vi "ActorDB-CheckIfPartExists.vi"(7 "Request Body":string, 8 "error in":errorcluster, 11 "Database-Actor in":refnum<class "PartCertDatabase-Actor.lvclass">) -> (0 "error out":errorcluster, 2 "Part number not found?":bool, 3 "Database-Actor out":refnum<class "PartCertDatabase-Actor.lvclass">)   [LabVIEW 2013, in "PartCertDatabase-Actor.lvclass"]
uses:
  PartCertDatabase-Actor.lvclass
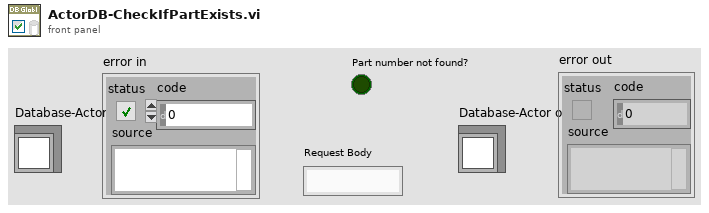
[diagram p1: front panel]
types:
  T1 = cluster{"Table":string, "SQL Statement":string, "Update All":bool, "Payload":string, "Reply Command":string, "Type Of Insertion":i32}
  T2 = cluster{"Manufacturing-Part Number":string, "Array of Cluster Data":cluster{"Label Instructions":string, "Path for Picture Label":path, "Path for Picture Label 2":path, "Path for Picture Label 3":path, "Path for Picture Label 4":path, "Path for Picture Label 5":path, "Path for Picture Label 6":path, "Path for Picture Label 7":path, "Label Instructions 2":string, "Label Instructions 3":string}[], "Type of Insert":i32}
  T3 = cluster{"Manufacturing-Part Number":string, "Step Number":dbl, "Gernal Cluster Data":cluster{"Label Instructions":string, "Path for Picture Label":path, "Path for Picture Label 2":path, "Path for Picture Label 3":path, "Path for Picture Label 4":path, "Path for Picture Label 5":path, "Path for Picture Label 6":path, "Path for Picture Label 7":path}, "Type of Insert":i32}
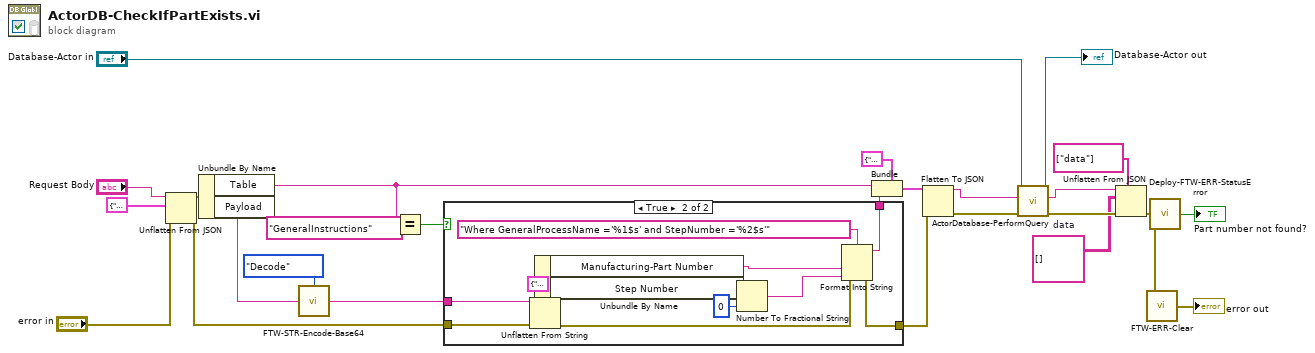
[diagram p0: block diagram]
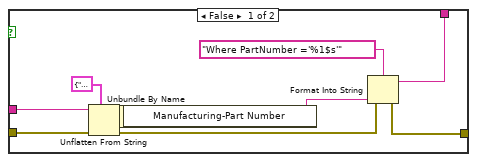
[diagram p2: hidden frame]
diagram:
  w7 = string[][] []  # data
  n1 = Unflatten From JSON(JSON string="Request Body", type and defaults=T1 {"Table"="", "SQL Statement"="", "Update All"=FALSE, "Payload"="", "Reply Command"="", "Type Of Insertion"=0} ("cluster"), error in (no error)="error in") -> (value=w23:T1, error out=w12:errorcluster)  [unwired: 4 in]
  n2 = Unbundle By Name(w23) -> ("Table"=w2:string, "Payload"=w21:string)
  n3 = call "FTW-STR-Encode-Base64.vi"("Input"=w21, "Direction"=enum16{"Encode", "Decode"}."Decode") -> ("Output"=w20:string)
  n4 = Equal?(x=w2, y="GeneralInstructions") -> (x = y?=w1:bool)
  n5 = case shown="True" w1 {
    tunnel: w20 -> [w35 w38]
    tunnel: [w30 w39] -> w17
    tunnel: [w29 w40] -> w16
    tunnel: w12 -> [w28 w41]
    frame False {
      n6 = Unflatten From String(type=T2 {"Manufacturing-Part Number"="", "Array of Cluster Data"=[], "Type of Insert"=0} ("cluster"), binary string=w35, error in (no error)=w28) -> (value=w33:T2, error out=w27:errorcluster)  [unwired: 2 in, 1 out]
      n7 = Unbundle By Name(w33) -> ("Manufacturing-Part Number"=w32:string)
      n8 = Format Into String(format string="Where PartNumber ='%1$s'" ("SQL Statement"), error in=w27, w32) -> (resulting string=w30:string, error out=w29:errorcluster)  [unwired: 1 in]
    }
    frame True {
      n9 = Unflatten From String(type=T3 {"Manufacturing-Part Number"="", "Step Number"=0.0, "Gernal Cluster Data"={"Label Instructions"="", "Path for Picture Label"=path "", "Path for Picture Label 2"=path "", "Path for Picture Label 3"=path "", "Path for Picture Label 4"=path "", "Path for Picture Label 5"=path "", "Path for Picture Label 6"=path "", "Path for Picture Label 7"=path ""}, "Type of Insert"=0} ("cluster"), binary string=w38, error in (no error)=w41) -> (value=w44:T3, error out=w42:errorcluster)  [unwired: 2 in, 1 out]
      n10 = Unbundle By Name(w44) -> ("Manufacturing-Part Number"=w43:string, "Step Number"=w46:dbl)
      n11 = Number To Fractional String(number=w46, precision (6)=i16 0) -> (F-format string=w47:string)  [unwired: 2 in]
      n12 = Format Into String(format string="Where GeneralProcessName ='%1$s' and StepNumber ='%2$s'" ("SQL Statement"), error in=w42, w43, w47) -> (resulting string=w39:string, error out=w40:errorcluster)  [unwired: 1 in]
    }
  }
  n13 = Bundle(cluster=cluster{"Table":string, "SQL Statement":string} {"Table"="", "SQL Statement"=""}, "Table"=w2, "SQL Statement"=w17) -> (w19:cluster{"Table":string, "SQL Statement":string})
  n14 = Flatten To JSON(anything=w19, error in (no error)=w16) -> (JSON string=w14:string, 11:w15:errorcluster)  [unwired: 1 in]
  n15 = call "ActorDatabase-PerformQuery.vi"("error in (no error)"=w15, "Payload from Actor"=w14, "Database-Actor in"="Database-Actor in") -> ("error out"=w10:errorcluster, "Payload To Actor"=w8:string, "Database-Actor out"=→"Database-Actor out":refnum<class "PartCertDatabase-Actor.lvclass">)  [unwired: 6 in]
  n16 = Unflatten From JSON(path=string[] ["data"], JSON string=w8, type and defaults=w7, error in (no error)=w10) -> (error out=w5:errorcluster)  [unwired: 3 in, 1 out]
  n17 = call "FTW-ERR-Clear.vi"("error to snuff"=w5) -> ("no error"=→"error out":errorcluster)
  n18 = call <resource>:"Deploy-FTW-ERR-StatusError.vi"("error to check"=w5) -> ("Error?"=→"Part number not found?":bool)
